vi "Unknown Error Code constant.vi"() -> (3 "Azure Unknown Error Code value":i32)   [LabVIEW 2015, in "NI_Azure_Core.lvlib"]
uses:
  NI_Azure_Core.lvlib
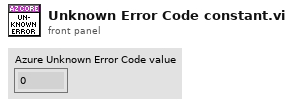
[diagram p1: front panel]
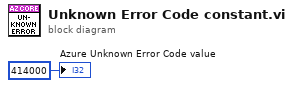
[diagram p0: block diagram]
diagram:
  "Azure Unknown Error Code value" <- 414000
